vi "Controlar motor.vi"() -> ()   [LabVIEW 2018]
panel:
  out "s? t:f":i32
  out "Numeric":dbl
  out "Waveform Chart":dbl(graph)
  in  "signo":bool
  in  "Amplitud":dbl(knob) scale=0.0..8.0
  in  "Ciclo de trabajo":dbl(knob) scale=0.0..100.0
  in  "Frecuencia":dbl(knob) scale=0.0..30.0
  in  "stop":bool
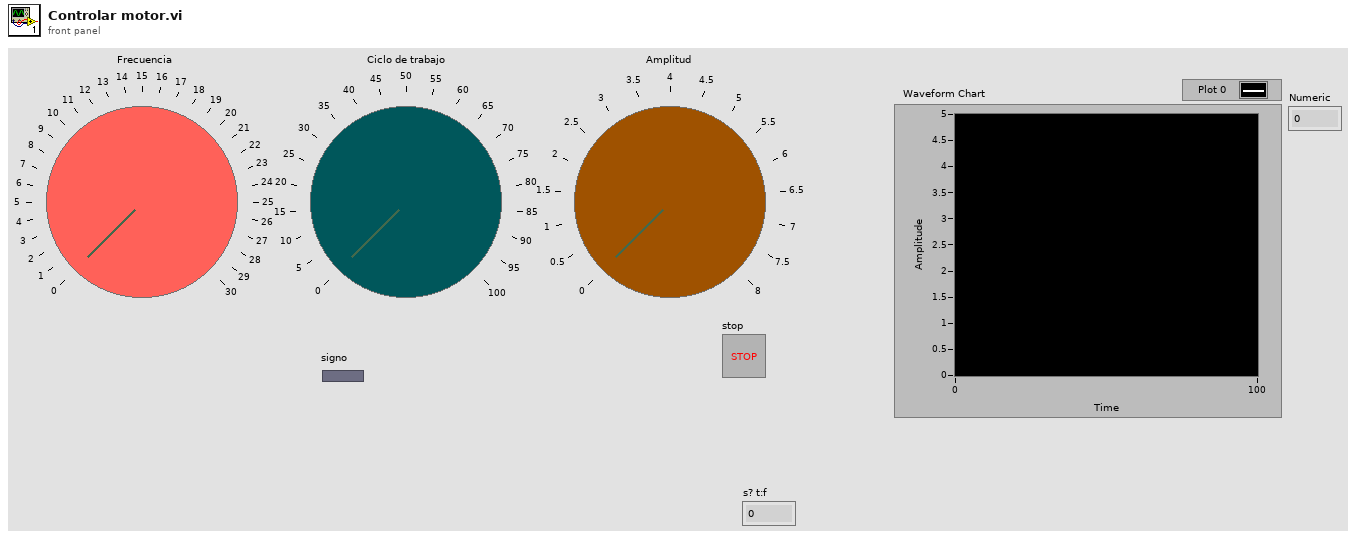
[diagram p1: front panel]
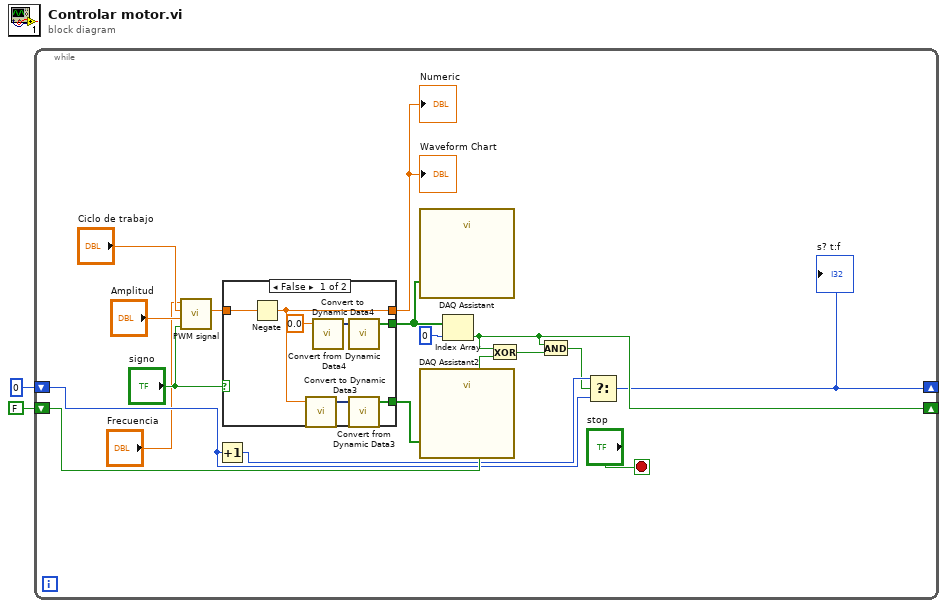
[diagram p0: block diagram]
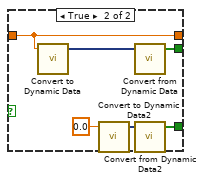
[diagram p2: hidden frame]
diagram:
  n1 = while {
    shift-right: [w8] -> _
    shift-left: FALSE -> [w10]
    shift-right: [w7] -> _
    shift-left: 0 -> [w6]
    stop <- "stop" stop-if-true
    n2 = call "PWM signal.vi"("Signo"="signo", "Amplitud"="Amplitud", "Ciclo de trabajo"="Ciclo de trabajo", "Frecuencia"="Frecuencia") -> ("Waveform Chart"=w18:dbl)  [unwired: 7 in]
    n3 = Increment(x=w6) -> (x+1=w5:i32)
    n4 = case shown="False" "signo" {
      tunnel: w18 -> [w21 w27]
      tunnel: [w23 w31] -> w12
      tunnel: [w25 w28] -> w15
      tunnel: [w20 w27] -> w13
      frame False {
        n5 = Negate(x=w21) -> (-x=w20:dbl)
        n6 = call "Convert to Dynamic Data3"("Double"=w20) -> ("Dynamic Data Type"=w26:dynamicdata)  [unwired: 3 in]
        n7 = call "Convert to Dynamic Data4"("Double"=0.0) -> ("Dynamic Data Type"=w24:dynamicdata)  [unwired: 3 in]
        n8 = call "Convert from Dynamic Data4"("Dynamic Data Type"=w24) -> ("Array"=w23:bool[])  [unwired: 3 in]
        n9 = call "Convert from Dynamic Data3"("Dynamic Data Type"=w26) -> ("Array"=w25:bool[])  [unwired: 3 in]
      }
      frame True {
        n10 = call "Convert to Dynamic Data"("Double"=w27) -> ("Dynamic Data Type"=w32:dynamicdata)  [unwired: 3 in]
        n11 = call "Convert to Dynamic Data2"("Double"=0.0) -> ("Dynamic Data Type"=w30:dynamicdata)  [unwired: 3 in]
        n12 = call "Convert from Dynamic Data"("Dynamic Data Type"=w32) -> ("Array"=w31:bool[])  [unwired: 3 in]
        n13 = call "Convert from Dynamic Data2"("Dynamic Data Type"=w30) -> ("Array"=w28:bool[])  [unwired: 3 in]
      }
    }
    "Numeric" <- w13
    "Waveform Chart" <- w13
    n14 = call "DAQ Assistant"("data"=w12) -> ()  [unwired: 17 in, 2 out]
    n15 = call "DAQ Assistant2"("data"=w15) -> ()  [unwired: 17 in, 2 out]
    n16 = Index Array(array=w12, index=0) -> (element=w8:bool)
    n17 = Exclusive Or(1:w10, 2:w8) -> (0:w9:bool)
    n18 = And(x=w8, y=w9) -> (x .and. y?=w3:bool)
    n19 = Select(t=w5, s=w3, f=w6) -> (s? t:f=w7:i32)
    "s? t:f" <- w7
  }
